vi "Game.vi"() -> ()   [LabVIEW 2019]
uses:
  Global 8.vi
panel:
  out "Ring":u16(ring)
  out "Ring 2":u16(ring)
  out "Ring 3":u16(ring)
  out "Ring 4":u16(ring)
  out "Ring 5":u16(ring)
  out "Ring 6":u16(ring)
  out "Ring 7":u16(ring)
  out "Ring 8":u16(ring)
  out "Ring 9":u16(ring)
  out "Ring 10":u16(ring)
  out "Ring 11":u16(ring)
  out "Ring 12":u16(ring)
  out "Ring 13":u16(ring)
  out "Ring 14":u16(ring)
  out "Ring 15":u16(ring)
  out "Ring 16":u16(ring)
  out "Ring 17":u16(ring)
  out "Ring 18":u16(ring)
  out "Ring 19":u16(ring)
  out "Ring 20":u16(ring)
  out "Ring 21":u16(ring)
  out "Ring 22":u16(ring)
  out "Ring 23":u16(ring)
  out "Ring 24":u16(ring)
  out "Ring 25":u16(ring)
  out "Ring 26":u16(ring)
  out "Ring 27":u16(ring)
  out "Ring 28":u16(ring)
  out "Ring 29":u16(ring)
  out "Ring 30":u16(ring)
  out "Ring 31":u16(ring)
  out "Ring 32":u16(ring)
  out "Ring 33":u16(ring)
  out "Ring 34":u16(ring)
  out "Ring 35":u16(ring)
  out "Ring 36":u16(ring)
  out "Ring 37":u16(ring)
  out "Ring 38":u16(ring)
  out "Ring 39":u16(ring)
  out "Ring 40":u16(ring)
  out "Ring 41":u16(ring)
  out "Ring 42":u16(ring)
  out "Ring 43":u16(ring)
  out "Ring 44":u16(ring)
  out "Ring 45":u16(ring)
  out "Ring 46":u16(ring)
  out "Ring 47":u16(ring)
  out "Ring 48":u16(ring)
  out "Ring 49":u16(ring)
  out "Ring 50":u16(ring)
  out "Ring 51":u16(ring)
  out "Ring 52":u16(ring)
  out "Ring 53":u16(ring)
  out "Ring 54":u16(ring)
  out "Ring 55":u16(ring)
  out "Ring 56":u16(ring)
  out "Ring 57":u16(ring)
  out "Ring 58":u16(ring)
  out "Ring 59":u16(ring)
  out "Ring 60":u16(ring)
  out "Ring 61":u16(ring)
  out "Ring 62":u16(ring)
  out "Ring 63":u16(ring)
  out "Ring 64":u16(ring)
  out "Ring 65":u16(ring)
  out "Ring 66":u16(ring)
  out "Ring 67":u16(ring)
  out "Ring 68":u16(ring)
  out "Ring 69":u16(ring)
  out "Ring 70":u16(ring)
  out "Ring 71":u16(ring)
  out "Ring 72":u16(ring)
  out "Ring 73":u16(ring)
  out "Ring 74":u16(ring)
  out "Ring 75":u16(ring)
  out "Ring 76":u16(ring)
  out "Ring 77":u16(ring)
  out "Ring 78":u16(ring)
  out "Ring 79":u16(ring)
  out "Ring 80":u16(ring)
  out "Ring 81":u16(ring)
  out "Ring 82":u16(ring)
  out "Ring 83":u16(ring)
  out "Ring 84":u16(ring)
  out "Ring 85":u16(ring)
  out "Ring 86":u16(ring)
  out "Ring 87":u16(ring)
  out "Ring 88":u16(ring)
  out "Ring 89":u16(ring)
  out "Ring 90":u16(ring)
  out "Ring 91":u16(ring)
  out "Ring 92":u16(ring)
  out "Ring 93":u16(ring)
  out "Ring 94":u16(ring)
  out "Ring 95":u16(ring)
  out "Ring 96":u16(ring)
  out "Ring 97":u16(ring)
  out "Ring 98":u16(ring)
  out "Ring 99":u16(ring)
  out "Ring 100":u16(ring)
  out "p4":dbl
  out "p3":dbl
  out "p2":dbl
  out "p1":dbl
  out "Boolean 4":bool
  out "Boolean 3":bool
  out "Boolean 2":bool
  out "Boolean":bool
  out "Player 1":string
  out "Player 2":string
  out "Player 3":string
  out "Player 4":string
  out "score 2":u16
  out "Dice 1":i32(ring)
  in  "Roll Button":bool
  out "score":u16
  in  "close":bool
  # "Player no."
  # "Score"
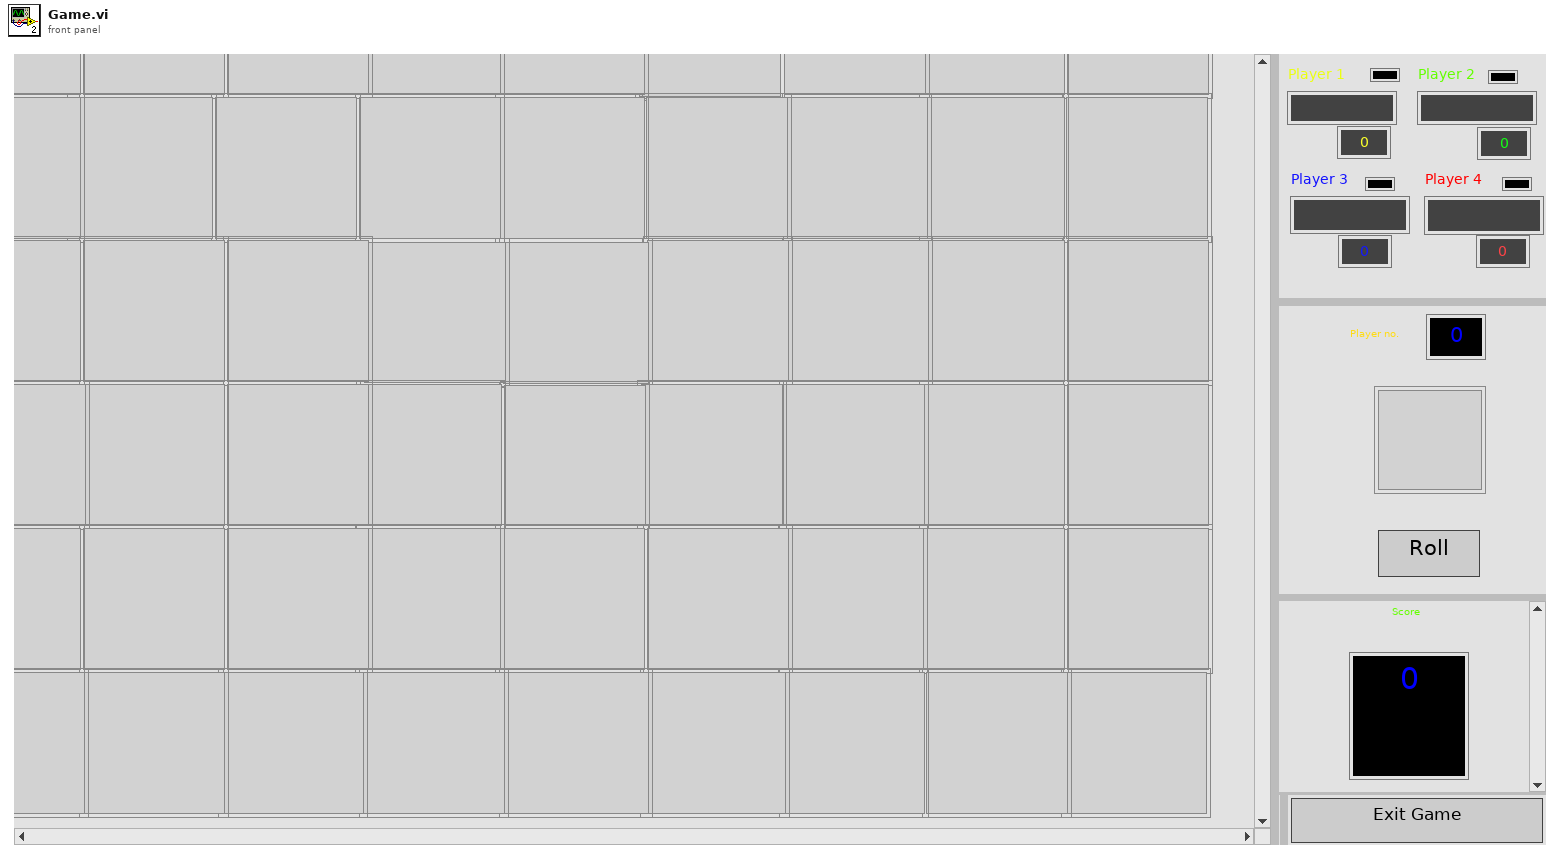
[diagram p1: front panel]
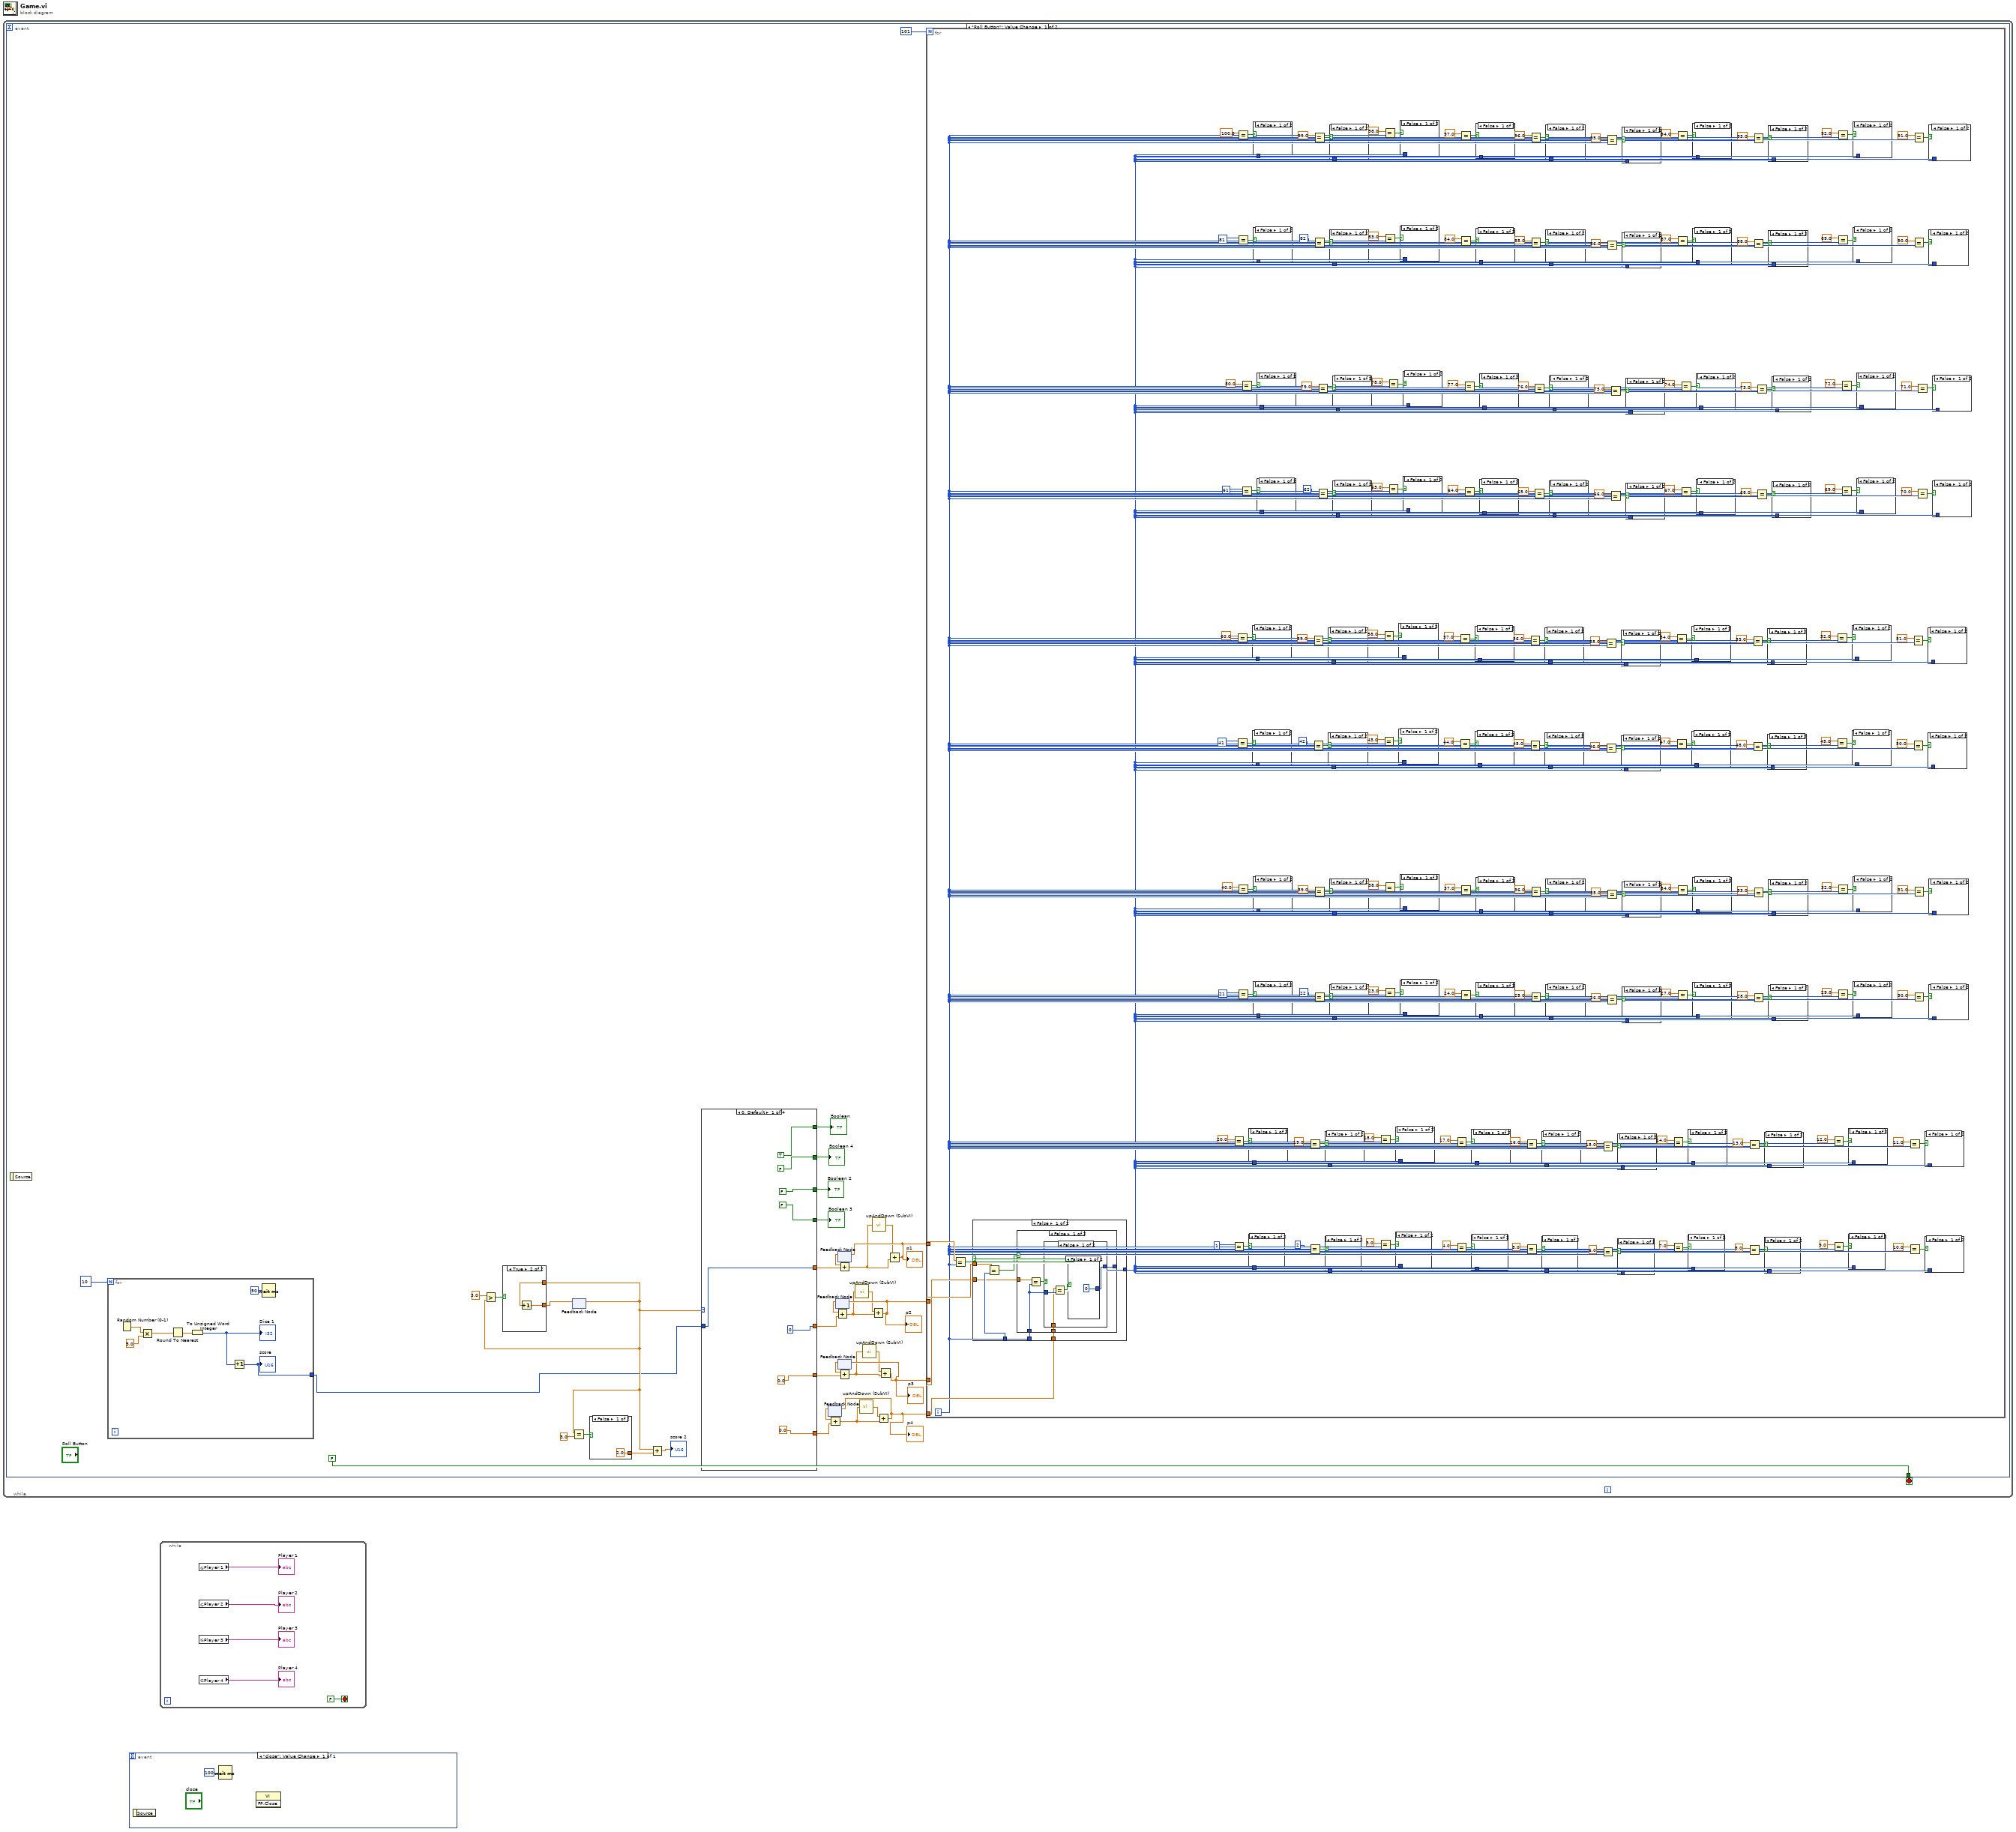
[diagram p0: block diagram]
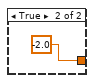
[diagram p2: hidden frame]
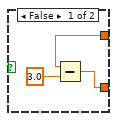
[diagram p3: hidden frame]
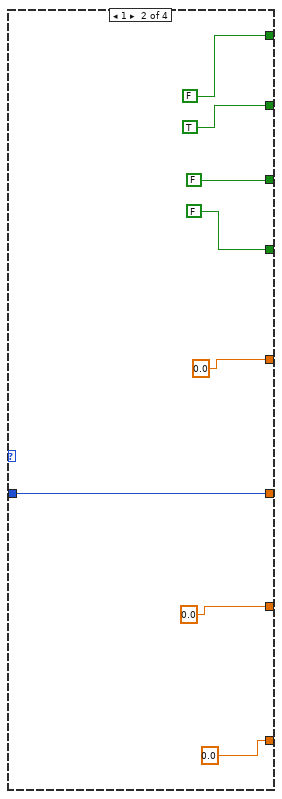
[diagram p4: hidden frame]
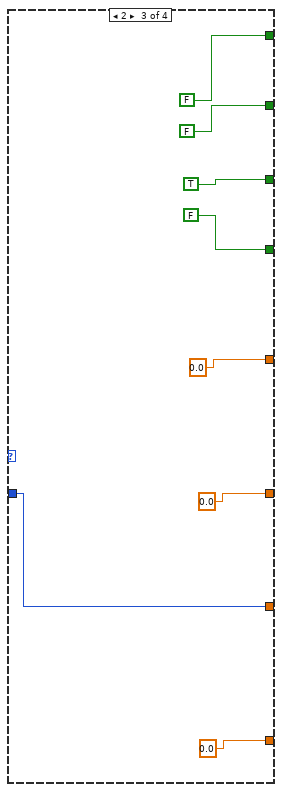
[diagram p5: hidden frame]
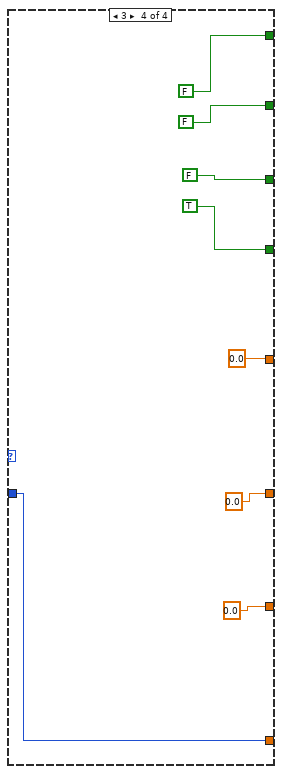
[diagram p6: hidden frame]
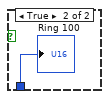
[diagram p7: hidden frame]
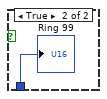
[diagram p8: hidden frame]
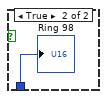
[diagram p9: hidden frame]
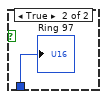
[diagram p10: hidden frame]
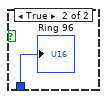
[diagram p11: hidden frame]
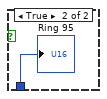
[diagram p12: hidden frame]
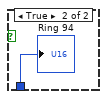
[diagram p13: hidden frame]
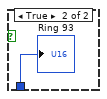
[diagram p14: hidden frame]
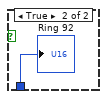
[diagram p15: hidden frame]
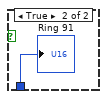
[diagram p16: hidden frame]
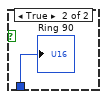
[diagram p17: hidden frame]
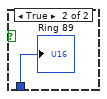
[diagram p18: hidden frame]
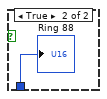
[diagram p19: hidden frame]
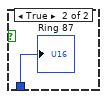
[diagram p20: hidden frame]
diagram:
  n1 = while {
    stop <- w1 stop-if-true
    n2 = event shown="[0] \"Roll Button\": Value Change" {
      selector: _ -> [_ _]
      dyn-events: _ -> [_ _]
      timeout: _ -> [_ _]
      tunnel: [FALSE TRUE] -> w1
      event "Roll Button": Value Change {
        n3 = event-data() -> ()  [unwired: 1 in, 1 out]
        n4 = for {
          N: 10 -> [_]
          tunnel: [w405] -> w2
          n5 = Random Number (0-1)() -> (number: 0 to 1=w410:dbl)
          n6 = Multiply(x=w410, y=5.0) -> (x*y=w408:dbl)
          n7 = Round To Nearest(number=w408) -> (nearest integer value=w407:dbl)
          n8 = To Unsigned Word Integer(number=w407) -> (unsigned 16bit integer=w406:u16)
          "Dice 1" <- w406
          n9 = Increment(x=w406) -> (x+1=w405:u16)
          "score" <- w405
          n10 = Wait (ms)(milliseconds to wait=u32 50) -> ()  [unwired: 1 out]
        }
        n11 = feedback #1() -> (w3:dbl)  [unwired: 1 in]
        n12 = Greater?(x=3.0, y=w3) -> (0:w26:bool)
        n13 = case shown="True" w26 {
          tunnel: [w42 w44] -> w24
          tunnel: w3 -> [w41 w43]
          frame False {
            n14 = Subtract(x=w41, y=3.0) -> (x-y=w42:dbl)
          }
          frame True {
            n15 = Increment(x=w43) -> (x+1=w44:dbl)
          }
        }
        n16 = feedback-in #1(w24) -> ()
        n17 = Equal?(x=w3, y=3.0) -> (x = y?=w18:bool)
        n18 = case shown="False" w18 {
          tunnel: [2.0 ("y") -2.0 ("y")] -> w16
          frame False {
          }
          frame True {
          }
        }
        n19 = Add(x=w3, y=w16) -> (x+y=→"score 2":dbl)
        n20 = case shown="0, Default" w3 {
          tunnel: [0 w59 0.0 ("y") 0.0 ("y")] -> w33
          tunnel: w2 -> [w51 w59 w68 w76]
          tunnel: [w51 0.0 ("y") 0.0 ("y") 0.0 ("y")] -> w32
          tunnel: [0.0 ("y") 0.0 ("y") w68 0.0 ("y")] -> w29
          tunnel: [0.0 ("y") 0.0 ("y") 0.0 ("y") w76] -> w28
          tunnel: [TRUE FALSE FALSE FALSE] -> w23
          tunnel: [FALSE TRUE FALSE FALSE] -> w22
          tunnel: [FALSE FALSE TRUE FALSE] -> w21
          tunnel: [FALSE FALSE FALSE TRUE] -> w20
          frame 0, Default {
          }
          frame 1 {
          }
          frame 2 {
          }
          frame 3 {
          }
        }
        "Boolean" <- w23
        "Boolean 2" <- w21
        "Boolean 3" <- w20
        "Boolean 4" <- w22
        n21 = feedback #2() -> (w30:dbl)  [unwired: 1 in]
        n22 = Add(x=w30, y=w28) -> (x+y=w4:dbl)
        n23 = feedback #3() -> (w34:dbl)  [unwired: 1 in]
        n24 = Add(x=w34, y=w33) -> (x+y=w10:dbl)
        n25 = feedback #4() -> (w35:dbl)  [unwired: 1 in]
        n26 = feedback #5() -> (w31:dbl)  [unwired: 1 in]
        n27 = Add(x=w35, y=w32) -> (x+y=w13:dbl)
        n28 = Add(x=w31, y=w29) -> (x+y=w7:dbl)
        n29 = call "upAndDown (SubVI).vi"("Numeric"=w10) -> ("Numeric 2"=w11:dbl)
        n30 = call "upAndDown (SubVI).vi"("Numeric"=w4) -> ("Numeric 2"=w6:dbl)
        n31 = call "upAndDown (SubVI).vi"("Numeric"=w7) -> ("Numeric 2"=w8:dbl)
        n32 = Add(x=w11, y=w10) -> (x+y=w12:dbl)
        "p2" <- w12
        n33 = feedback-in #3(w12) -> ()
        n34 = call "upAndDown (SubVI).vi"("Numeric"=w13) -> ("Numeric 2"=w14:dbl)
        n35 = Add(x=w6, y=w4) -> (x+y=w5:dbl)
        "p4" <- w5
        n36 = feedback-in #2(w5) -> ()
        n37 = Add(x=w8, y=w7) -> (x+y=w9:dbl)
        "p3" <- w9
        n38 = feedback-in #5(w9) -> ()
        n39 = Add(x=w14, y=w13) -> (x+y=w15:dbl)
        "p1" <- w15
        n40 = feedback-in #4(w15) -> ()
        n41 = for {
          N: 101 -> [_]
          tunnel: w15 -> [w242]
          tunnel: w12 -> [w241]
          tunnel: w9 -> [w240]
          tunnel: w5 -> [w239]
          i -> [w78]
          n42 = Equal?(x=w242, y=w78) -> (x = y?=w243:bool)
          n43 = case shown="False" w243 {
            tunnel: [w369 1] -> w77
            tunnel: w78 -> [w368 _]
            tunnel: w241 -> [w370 _]
            tunnel: w78 -> [w366 _]
            tunnel: w240 -> [w365 _]
            tunnel: w239 -> [w364 _]
            frame False {
              n44 = Equal?(x=w370, y=w368) -> (x = y?=w367:bool)
              n45 = case shown="False" w367 {
                tunnel: [w375 2] -> w369
                tunnel: w366 -> [w372 _]
                tunnel: w365 -> [w373 _]
                tunnel: w364 -> [w371 _]
                frame False {
                  n46 = Equal?(x=w373, y=w372) -> (x = y?=w374:bool)
                  n47 = case shown="False" w374 {
                    tunnel: [w376 3] -> w375
                    tunnel: w372 -> [w378 _]
                    tunnel: w371 -> [w377 _]
                    frame False {
                      n48 = Equal?(x=w377, y=w378) -> (x = y?=w379:bool)
                      n49 = case shown="False" w379 {
                        tunnel: [0 4] -> w376
                        frame False {
                        }
                        frame True {
                        }
                      }
                    }
                    frame True {
                    }
                  }
                }
                frame True {
                }
              }
            }
            frame True {
            }
          }
          n50 = Equal?(x=20.0, y=w78) -> (x = y?=w265:bool)
          n51 = Equal?(x=1, y=w78) -> (x = y?=w283:bool)
          n52 = Equal?(x=60.0, y=w78) -> (x = y?=w180:bool)
          n53 = Equal?(x=41, y=w78) -> (x = y?=w198:bool)
          n54 = Equal?(x=100.0, y=w78) -> (x = y?=w100:bool)
          n55 = Equal?(x=81, y=w78) -> (x = y?=w118:bool)
          n56 = Equal?(x=40.0, y=w78) -> (x = y?=w220:bool)
          n57 = Equal?(x=21, y=w78) -> (x = y?=w238:bool)
          n58 = Equal?(x=80.0, y=w78) -> (x = y?=w140:bool)
          n59 = Equal?(x=61, y=w78) -> (x = y?=w158:bool)
          n60 = case shown="False" w265 {
            tunnel: w77 -> [_ w394]
            frame False {
            }
            frame True {
              "Ring 11" <- w394
            }
          }
          n61 = case shown="False" w283 {
            tunnel: w77 -> [_ w404]
            frame False {
            }
            frame True {
              "Ring" <- w404
            }
          }
          n62 = case shown="False" w180 {
            tunnel: w77 -> [_ w333]
            frame False {
            }
            frame True {
              "Ring 51" <- w333
            }
          }
          n63 = case shown="False" w198 {
            tunnel: w77 -> [_ w343]
            frame False {
            }
            frame True {
              "Ring 41" <- w343
            }
          }
          n64 = case shown="False" w100 {
            tunnel: w77 -> [_ w293]
            frame False {
            }
            frame True {
              "Ring 91" <- w293
            }
          }
          n65 = case shown="False" w118 {
            tunnel: w77 -> [_ w303]
            frame False {
            }
            frame True {
              "Ring 81" <- w303
            }
          }
          n66 = case shown="False" w220 {
            tunnel: w77 -> [_ w353]
            frame False {
            }
            frame True {
              "Ring 31" <- w353
            }
          }
          n67 = case shown="False" w238 {
            tunnel: w77 -> [_ w363]
            frame False {
            }
            frame True {
              "Ring 21" <- w363
            }
          }
          n68 = case shown="False" w140 {
            tunnel: w77 -> [_ w313]
            frame False {
            }
            frame True {
              "Ring 71" <- w313
            }
          }
          n69 = case shown="False" w158 {
            tunnel: w77 -> [_ w323]
            frame False {
            }
            frame True {
              "Ring 61" <- w323
            }
          }
          n70 = Equal?(x=19.0, y=w78) -> (x = y?=w263:bool)
          n71 = Equal?(x=2, y=w78) -> (x = y?=w282:bool)
          n72 = Equal?(x=59.0, y=w78) -> (x = y?=w178:bool)
          n73 = Equal?(x=42, y=w78) -> (x = y?=w197:bool)
          n74 = Equal?(x=99.0, y=w78) -> (x = y?=w98:bool)
          n75 = Equal?(x=82, y=w78) -> (x = y?=w117:bool)
          n76 = Equal?(x=39.0, y=w78) -> (x = y?=w218:bool)
          n77 = Equal?(x=22, y=w78) -> (x = y?=w237:bool)
          n78 = Equal?(x=79.0, y=w78) -> (x = y?=w138:bool)
          n79 = Equal?(x=62, y=w78) -> (x = y?=w157:bool)
          n80 = case shown="False" w263 {
            tunnel: w77 -> [_ w393]
            frame False {
            }
            frame True {
              "Ring 12" <- w393
            }
          }
          n81 = case shown="False" w282 {
            tunnel: w77 -> [_ w403]
            frame False {
            }
            frame True {
              "Ring 2" <- w403
            }
          }
          n82 = case shown="False" w178 {
            tunnel: w77 -> [_ w332]
            frame False {
            }
            frame True {
              "Ring 52" <- w332
            }
          }
          n83 = case shown="False" w197 {
            tunnel: w77 -> [_ w342]
            frame False {
            }
            frame True {
              "Ring 42" <- w342
            }
          }
          n84 = case shown="False" w98 {
            tunnel: w77 -> [_ w292]
            frame False {
            }
            frame True {
              "Ring 92" <- w292
            }
          }
          n85 = case shown="False" w117 {
            tunnel: w77 -> [_ w302]
            frame False {
            }
            frame True {
              "Ring 82" <- w302
            }
          }
          n86 = case shown="False" w218 {
            tunnel: w77 -> [_ w352]
            frame False {
            }
            frame True {
              "Ring 32" <- w352
            }
          }
          n87 = case shown="False" w237 {
            tunnel: w77 -> [_ w362]
            frame False {
            }
            frame True {
              "Ring 22" <- w362
            }
          }
          n88 = case shown="False" w138 {
            tunnel: w77 -> [_ w312]
            frame False {
            }
            frame True {
              "Ring 72" <- w312
            }
          }
          n89 = case shown="False" w157 {
            tunnel: w77 -> [_ w322]
            frame False {
            }
            frame True {
              "Ring 62" <- w322
            }
          }
          n90 = Equal?(x=18.0, y=w78) -> (x = y?=w261:bool)
          n91 = Equal?(x=3.0, y=w78) -> (x = y?=w281:bool)
          n92 = Equal?(x=58.0, y=w78) -> (x = y?=w176:bool)
          n93 = Equal?(x=43.0, y=w78) -> (x = y?=w196:bool)
          n94 = Equal?(x=98.0, y=w78) -> (x = y?=w96:bool)
          n95 = Equal?(x=83.0, y=w78) -> (x = y?=w116:bool)
          n96 = Equal?(x=38.0, y=w78) -> (x = y?=w216:bool)
          n97 = Equal?(x=23.0, y=w78) -> (x = y?=w236:bool)
          n98 = Equal?(x=78.0, y=w78) -> (x = y?=w136:bool)
          n99 = Equal?(x=63.0, y=w78) -> (x = y?=w156:bool)
          n100 = case shown="False" w261 {
            tunnel: w77 -> [_ w392]
            frame False {
            }
            frame True {
              "Ring 13" <- w392
            }
          }
          n101 = case shown="False" w281 {
            tunnel: w77 -> [_ w402]
            frame False {
            }
            frame True {
              "Ring 3" <- w402
            }
          }
          n102 = case shown="False" w176 {
            tunnel: w77 -> [_ w331]
            frame False {
            }
            frame True {
              "Ring 53" <- w331
            }
          }
          n103 = case shown="False" w196 {
            tunnel: w77 -> [_ w341]
            frame False {
            }
            frame True {
              "Ring 43" <- w341
            }
          }
          n104 = case shown="False" w96 {
            tunnel: w77 -> [_ w291]
            frame False {
            }
            frame True {
              "Ring 93" <- w291
            }
          }
          n105 = case shown="False" w116 {
            tunnel: w77 -> [_ w301]
            frame False {
            }
            frame True {
              "Ring 83" <- w301
            }
          }
          n106 = case shown="False" w216 {
            tunnel: w77 -> [_ w351]
            frame False {
            }
            frame True {
              "Ring 33" <- w351
            }
          }
          n107 = case shown="False" w236 {
            tunnel: w77 -> [_ w361]
            frame False {
            }
            frame True {
              "Ring 23" <- w361
            }
          }
          n108 = case shown="False" w136 {
            tunnel: w77 -> [_ w311]
            frame False {
            }
            frame True {
              "Ring 73" <- w311
            }
          }
          n109 = case shown="False" w156 {
            tunnel: w77 -> [_ w321]
            frame False {
            }
            frame True {
              "Ring 63" <- w321
            }
          }
          n110 = Equal?(x=17.0, y=w78) -> (x = y?=w259:bool)
          n111 = Equal?(x=4.0, y=w78) -> (x = y?=w279:bool)
          n112 = Equal?(x=57.0, y=w78) -> (x = y?=w174:bool)
          n113 = Equal?(x=44.0, y=w78) -> (x = y?=w194:bool)
          n114 = Equal?(x=97.0, y=w78) -> (x = y?=w94:bool)
          n115 = Equal?(x=84.0, y=w78) -> (x = y?=w114:bool)
          n116 = Equal?(x=37.0, y=w78) -> (x = y?=w214:bool)
          n117 = Equal?(x=24.0, y=w78) -> (x = y?=w234:bool)
          n118 = Equal?(x=77.0, y=w78) -> (x = y?=w134:bool)
          n119 = Equal?(x=64.0, y=w78) -> (x = y?=w154:bool)
          n120 = case shown="False" w259 {
            tunnel: w77 -> [_ w391]
            frame False {
            }
            frame True {
              "Ring 14" <- w391
            }
          }
          n121 = case shown="False" w279 {
            tunnel: w77 -> [_ w401]
            frame False {
            }
            frame True {
              "Ring 4" <- w401
            }
          }
          n122 = case shown="False" w174 {
            tunnel: w77 -> [_ w330]
            frame False {
            }
            frame True {
              "Ring 54" <- w330
            }
          }
          n123 = case shown="False" w194 {
            tunnel: w77 -> [_ w340]
            frame False {
            }
            frame True {
              "Ring 44" <- w340
            }
          }
          n124 = case shown="False" w94 {
            tunnel: w77 -> [_ w290]
            frame False {
            }
            frame True {
              "Ring 94" <- w290
            }
          }
          n125 = case shown="False" w114 {
            tunnel: w77 -> [_ w300]
            frame False {
            }
            frame True {
              "Ring 84" <- w300
            }
          }
          n126 = case shown="False" w214 {
            tunnel: w77 -> [_ w350]
            frame False {
            }
            frame True {
              "Ring 34" <- w350
            }
          }
          n127 = case shown="False" w234 {
            tunnel: w77 -> [_ w360]
            frame False {
            }
            frame True {
              "Ring 24" <- w360
            }
          }
          n128 = case shown="False" w134 {
            tunnel: w77 -> [_ w310]
            frame False {
            }
            frame True {
              "Ring 74" <- w310
            }
          }
          n129 = case shown="False" w154 {
            tunnel: w77 -> [_ w320]
            frame False {
            }
            frame True {
              "Ring 64" <- w320
            }
          }
          n130 = Equal?(x=16.0, y=w78) -> (x = y?=w257:bool)
          n131 = Equal?(x=5.0, y=w78) -> (x = y?=w277:bool)
          n132 = Equal?(x=56.0, y=w78) -> (x = y?=w172:bool)
          n133 = Equal?(x=45.0, y=w78) -> (x = y?=w192:bool)
          n134 = Equal?(x=96.0, y=w78) -> (x = y?=w92:bool)
          n135 = Equal?(x=85.0, y=w78) -> (x = y?=w112:bool)
          n136 = Equal?(x=36.0, y=w78) -> (x = y?=w212:bool)
          n137 = Equal?(x=25.0, y=w78) -> (x = y?=w232:bool)
          n138 = Equal?(x=76.0, y=w78) -> (x = y?=w132:bool)
          n139 = Equal?(x=65.0, y=w78) -> (x = y?=w152:bool)
          n140 = case shown="False" w257 {
            tunnel: w77 -> [_ w390]
            frame False {
            }
            frame True {
              "Ring 15" <- w390
            }
          }
          n141 = case shown="False" w277 {
            tunnel: w77 -> [_ w400]
            frame False {
            }
            frame True {
              "Ring 5" <- w400
            }
          }
          n142 = case shown="False" w172 {
            tunnel: w77 -> [_ w329]
            frame False {
            }
            frame True {
              "Ring 55" <- w329
            }
          }
          n143 = case shown="False" w192 {
            tunnel: w77 -> [_ w339]
            frame False {
            }
            frame True {
              "Ring 45" <- w339
            }
          }
          n144 = case shown="False" w92 {
            tunnel: w77 -> [_ w289]
            frame False {
            }
            frame True {
              "Ring 95" <- w289
            }
          }
          n145 = case shown="False" w112 {
            tunnel: w77 -> [_ w299]
            frame False {
            }
            frame True {
              "Ring 85" <- w299
            }
          }
          n146 = case shown="False" w212 {
            tunnel: w77 -> [_ w349]
            frame False {
            }
            frame True {
              "Ring 35" <- w349
            }
          }
          n147 = case shown="False" w232 {
            tunnel: w77 -> [_ w359]
            frame False {
            }
            frame True {
              "Ring 25" <- w359
            }
          }
          n148 = case shown="False" w132 {
            tunnel: w77 -> [_ w309]
            frame False {
            }
            frame True {
              "Ring 75" <- w309
            }
          }
          n149 = case shown="False" w152 {
            tunnel: w77 -> [_ w319]
            frame False {
            }
            frame True {
              "Ring 65" <- w319
            }
          }
          n150 = Equal?(x=15.0, y=w78) -> (x = y?=w255:bool)
          n151 = Equal?(x=6.0, y=w78) -> (x = y?=w275:bool)
          n152 = Equal?(x=55.0, y=w78) -> (x = y?=w170:bool)
          n153 = Equal?(x=46.0, y=w78) -> (x = y?=w190:bool)
          n154 = Equal?(x=95.0, y=w78) -> (x = y?=w90:bool)
          n155 = Equal?(x=86.0, y=w78) -> (x = y?=w110:bool)
          n156 = Equal?(x=35.0, y=w78) -> (x = y?=w210:bool)
          n157 = Equal?(x=26.0, y=w78) -> (x = y?=w230:bool)
          n158 = Equal?(x=75.0, y=w78) -> (x = y?=w130:bool)
          n159 = Equal?(x=66.0, y=w78) -> (x = y?=w150:bool)
          n160 = case shown="False" w255 {
            tunnel: w77 -> [_ w389]
            frame False {
            }
            frame True {
              "Ring 16" <- w389
            }
          }
          n161 = case shown="False" w275 {
            tunnel: w77 -> [_ w399]
            frame False {
            }
            frame True {
              "Ring 6" <- w399
            }
          }
          n162 = case shown="False" w170 {
            tunnel: w77 -> [_ w328]
            frame False {
            }
            frame True {
              "Ring 56" <- w328
            }
          }
          n163 = case shown="False" w190 {
            tunnel: w77 -> [_ w338]
            frame False {
            }
            frame True {
              "Ring 46" <- w338
            }
          }
          n164 = case shown="False" w90 {
            tunnel: w77 -> [_ w288]
            frame False {
            }
            frame True {
              "Ring 96" <- w288
            }
          }
          n165 = case shown="False" w110 {
            tunnel: w77 -> [_ w298]
            frame False {
            }
            frame True {
              "Ring 86" <- w298
            }
          }
          n166 = case shown="False" w210 {
            tunnel: w77 -> [_ w348]
            frame False {
            }
            frame True {
              "Ring 36" <- w348
            }
          }
          n167 = case shown="False" w230 {
            tunnel: w77 -> [_ w358]
            frame False {
            }
            frame True {
              "Ring 26" <- w358
            }
          }
          n168 = case shown="False" w130 {
            tunnel: w77 -> [_ w308]
            frame False {
            }
            frame True {
              "Ring 76" <- w308
            }
          }
          n169 = case shown="False" w150 {
            tunnel: w77 -> [_ w318]
            frame False {
            }
            frame True {
              "Ring 66" <- w318
            }
          }
          n170 = Equal?(x=14.0, y=w78) -> (x = y?=w253:bool)
          n171 = Equal?(x=7.0, y=w78) -> (x = y?=w273:bool)
          n172 = Equal?(x=54.0, y=w78) -> (x = y?=w168:bool)
          n173 = Equal?(x=47.0, y=w78) -> (x = y?=w188:bool)
          n174 = Equal?(x=94.0, y=w78) -> (x = y?=w88:bool)
          n175 = Equal?(x=87.0, y=w78) -> (x = y?=w108:bool)
          n176 = Equal?(x=34.0, y=w78) -> (x = y?=w208:bool)
          n177 = Equal?(x=27.0, y=w78) -> (x = y?=w228:bool)
          n178 = Equal?(x=74.0, y=w78) -> (x = y?=w128:bool)
          n179 = Equal?(x=67.0, y=w78) -> (x = y?=w148:bool)
          n180 = case shown="False" w253 {
            tunnel: w77 -> [_ w388]
            frame False {
            }
            frame True {
              "Ring 17" <- w388
            }
          }
          n181 = case shown="False" w273 {
            tunnel: w77 -> [_ w398]
            frame False {
            }
            frame True {
              "Ring 7" <- w398
            }
          }
          n182 = case shown="False" w168 {
            tunnel: w77 -> [_ w327]
            frame False {
            }
            frame True {
              "Ring 57" <- w327
            }
          }
          n183 = case shown="False" w188 {
            tunnel: w77 -> [_ w337]
            frame False {
            }
            frame True {
              "Ring 47" <- w337
            }
          }
          n184 = case shown="False" w88 {
            tunnel: w77 -> [_ w287]
            frame False {
            }
            frame True {
              "Ring 97" <- w287
            }
          }
          n185 = case shown="False" w108 {
            tunnel: w77 -> [_ w297]
            frame False {
            }
            frame True {
              "Ring 87" <- w297
            }
          }
          n186 = case shown="False" w208 {
            tunnel: w77 -> [_ w347]
            frame False {
            }
            frame True {
              "Ring 37" <- w347
            }
          }
          n187 = case shown="False" w228 {
            tunnel: w77 -> [_ w357]
            frame False {
            }
            frame True {
              "Ring 27" <- w357
            }
          }
          n188 = case shown="False" w128 {
            tunnel: w77 -> [_ w307]
            frame False {
            }
            frame True {
              "Ring 77" <- w307
            }
          }
          n189 = case shown="False" w148 {
            tunnel: w77 -> [_ w317]
            frame False {
            }
            frame True {
              "Ring 67" <- w317
            }
          }
          n190 = Equal?(x=13.0, y=w78) -> (x = y?=w251:bool)
          n191 = Equal?(x=8.0, y=w78) -> (x = y?=w271:bool)
          n192 = Equal?(x=53.0, y=w78) -> (x = y?=w166:bool)
          n193 = Equal?(x=48.0, y=w78) -> (x = y?=w186:bool)
          n194 = Equal?(x=93.0, y=w78) -> (x = y?=w86:bool)
          n195 = Equal?(x=88.0, y=w78) -> (x = y?=w106:bool)
          n196 = Equal?(x=33.0, y=w78) -> (x = y?=w206:bool)
          n197 = Equal?(x=28.0, y=w78) -> (x = y?=w226:bool)
          n198 = Equal?(x=73.0, y=w78) -> (x = y?=w126:bool)
          n199 = Equal?(x=68.0, y=w78) -> (x = y?=w146:bool)
          n200 = case shown="False" w251 {
            tunnel: w77 -> [_ w387]
            frame False {
            }
            frame True {
              "Ring 18" <- w387
            }
          }
          n201 = case shown="False" w271 {
            tunnel: w77 -> [_ w397]
            frame False {
            }
            frame True {
              "Ring 8" <- w397
            }
          }
          n202 = case shown="False" w166 {
            tunnel: w77 -> [_ w326]
            frame False {
            }
            frame True {
              "Ring 58" <- w326
            }
          }
          n203 = case shown="False" w186 {
            tunnel: w77 -> [_ w336]
            frame False {
            }
            frame True {
              "Ring 48" <- w336
            }
          }
          n204 = case shown="False" w86 {
            tunnel: w77 -> [_ w286]
            frame False {
            }
            frame True {
              "Ring 98" <- w286
            }
          }
          n205 = case shown="False" w106 {
            tunnel: w77 -> [_ w296]
            frame False {
            }
            frame True {
              "Ring 88" <- w296
            }
          }
          n206 = case shown="False" w206 {
            tunnel: w77 -> [_ w346]
            frame False {
            }
            frame True {
              "Ring 38" <- w346
            }
          }
          n207 = case shown="False" w226 {
            tunnel: w77 -> [_ w356]
            frame False {
            }
            frame True {
              "Ring 28" <- w356
            }
          }
          n208 = case shown="False" w126 {
            tunnel: w77 -> [_ w306]
            frame False {
            }
            frame True {
              "Ring 78" <- w306
            }
          }
          n209 = case shown="False" w146 {
            tunnel: w77 -> [_ w316]
            frame False {
            }
            frame True {
              "Ring 68" <- w316
            }
          }
          n210 = Equal?(x=12.0, y=w78) -> (x = y?=w249:bool)
          n211 = Equal?(x=9.0, y=w78) -> (x = y?=w269:bool)
          n212 = Equal?(x=52.0, y=w78) -> (x = y?=w164:bool)
          n213 = Equal?(x=49.0, y=w78) -> (x = y?=w184:bool)
          n214 = Equal?(x=92.0, y=w78) -> (x = y?=w84:bool)
          n215 = Equal?(x=89.0, y=w78) -> (x = y?=w104:bool)
          n216 = Equal?(x=32.0, y=w78) -> (x = y?=w204:bool)
          n217 = Equal?(x=29.0, y=w78) -> (x = y?=w224:bool)
          n218 = Equal?(x=72.0, y=w78) -> (x = y?=w124:bool)
          n219 = Equal?(x=69.0, y=w78) -> (x = y?=w144:bool)
          n220 = case shown="False" w249 {
            tunnel: w77 -> [_ w386]
            frame False {
            }
            frame True {
              "Ring 19" <- w386
            }
          }
          n221 = case shown="False" w269 {
            tunnel: w77 -> [_ w396]
            frame False {
            }
            frame True {
              "Ring 9" <- w396
            }
          }
          n222 = case shown="False" w164 {
            tunnel: w77 -> [_ w325]
            frame False {
            }
            frame True {
              "Ring 59" <- w325
            }
          }
          n223 = case shown="False" w184 {
            tunnel: w77 -> [_ w335]
            frame False {
            }
            frame True {
              "Ring 49" <- w335
            }
          }
          n224 = case shown="False" w84 {
            tunnel: w77 -> [_ w285]
            frame False {
            }
            frame True {
              "Ring 99" <- w285
            }
          }
          n225 = case shown="False" w104 {
            tunnel: w77 -> [_ w295]
            frame False {
            }
            frame True {
              "Ring 89" <- w295
            }
          }
          n226 = case shown="False" w204 {
            tunnel: w77 -> [_ w345]
            frame False {
            }
            frame True {
              "Ring 39" <- w345
            }
          }
          n227 = case shown="False" w224 {
            tunnel: w77 -> [_ w355]
            frame False {
            }
            frame True {
              "Ring 29" <- w355
            }
          }
          n228 = case shown="False" w124 {
            tunnel: w77 -> [_ w305]
            frame False {
            }
            frame True {
              "Ring 79" <- w305
            }
          }
          n229 = case shown="False" w144 {
            tunnel: w77 -> [_ w315]
            frame False {
            }
            frame True {
              "Ring 69" <- w315
            }
          }
          n230 = Equal?(x=11.0, y=w78) -> (x = y?=w247:bool)
          n231 = Equal?(x=10.0, y=w78) -> (x = y?=w267:bool)
          n232 = Equal?(x=51.0, y=w78) -> (x = y?=w162:bool)
          n233 = Equal?(x=50.0, y=w78) -> (x = y?=w182:bool)
          n234 = Equal?(x=91.0, y=w78) -> (x = y?=w82:bool)
          n235 = Equal?(x=90.0, y=w78) -> (x = y?=w102:bool)
          n236 = Equal?(x=31.0, y=w78) -> (x = y?=w202:bool)
          n237 = Equal?(x=30.0, y=w78) -> (x = y?=w222:bool)
          n238 = Equal?(x=71.0, y=w78) -> (x = y?=w122:bool)
          n239 = Equal?(x=70.0, y=w78) -> (x = y?=w142:bool)
          n240 = case shown="False" w247 {
            tunnel: w77 -> [_ w385]
            frame False {
            }
            frame True {
              "Ring 20" <- w385
            }
          }
          n241 = case shown="False" w267 {
            tunnel: w77 -> [_ w395]
            frame False {
            }
            frame True {
              "Ring 10" <- w395
            }
          }
          n242 = case shown="False" w162 {
            tunnel: w77 -> [_ w324]
            frame False {
            }
            frame True {
              "Ring 60" <- w324
            }
          }
          n243 = case shown="False" w182 {
            tunnel: w77 -> [_ w334]
            frame False {
            }
            frame True {
              "Ring 50" <- w334
            }
          }
          n244 = case shown="False" w82 {
            tunnel: w77 -> [_ w284]
            frame False {
            }
            frame True {
              "Ring 100" <- w284
            }
          }
          n245 = case shown="False" w102 {
            tunnel: w77 -> [_ w294]
            frame False {
            }
            frame True {
              "Ring 90" <- w294
            }
          }
          n246 = case shown="False" w202 {
            tunnel: w77 -> [_ w344]
            frame False {
            }
            frame True {
              "Ring 40" <- w344
            }
          }
          n247 = case shown="False" w222 {
            tunnel: w77 -> [_ w354]
            frame False {
            }
            frame True {
              "Ring 30" <- w354
            }
          }
          n248 = case shown="False" w122 {
            tunnel: w77 -> [_ w304]
            frame False {
            }
            frame True {
              "Ring 80" <- w304
            }
          }
          n249 = case shown="False" w142 {
            tunnel: w77 -> [_ w314]
            frame False {
            }
            frame True {
              "Ring 70" <- w314
            }
          }
        }
      }
      event Timeout {
        n250 = event-data() -> ()  [unwired: 1 in, 3 out]
        n251 = One Button Dialog(message="Time out", button name ("OK")="Ok") -> ()  [unwired: 1 out]
      }
    }
  }
  n252 = event shown="[0] \"close\": Value Change" {
    selector: _ -> [_]
    dyn-events: _ -> [_]
    timeout: _ -> [_]
    event "close": Value Change {
      n253 = event-data() -> ()  [unwired: 1 in, 1 out]
      n254 = Wait (ms)(milliseconds to wait=u32 100) -> ()  [unwired: 1 out]
      n255 = invoke class="VI" method="FP.Close"() -> ()  [unwired: 3 in, 3 out]
    }
  }
  n256 = while {
    stop <- FALSE stop-if-true
    n257 = global read "Global 8.vi" "Player 1"() -> (→"Player 1":string)
    n258 = global read "Global 8.vi" "Player 2"() -> (→"Player 2":string)
    n259 = global read "Global 8.vi" "Player 3"() -> (→"Player 3":string)
    n260 = global read "Global 8.vi" "Player 4"() -> (→"Player 4":string)
  }
